vi "Constants.vi"() -> (1 "HelperProject path":path, 2 "HelperExecutable path":path, 3 "HelperMain path":path)   [LabVIEW 2016, in "DronaTest.lvlib"]
uses:
  DronaTest.lvlib
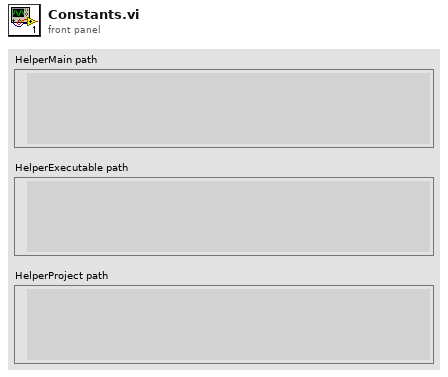
[diagram p1: front panel]
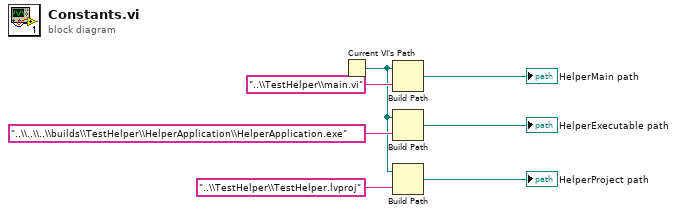
[diagram p0: block diagram]
diagram:
  n1 = Current VI's Path() -> (path=w2:path)
  n2 = Build Path(base path=w2, name or relative path="..\\TestHelper\\main.vi") -> (appended path=→"HelperMain path":path)
  n3 = Build Path(base path=w2, name or relative path="..\\..\\..\\builds\\TestHelper\\HelperApplication\\HelperApplication.exe") -> (appended path=→"HelperExecutable path":path)
  n4 = Build Path(base path=w2, name or relative path="..\\TestHelper\\TestHelper.lvproj") -> (appended path=→"HelperProject path":path)
